vi "filter channels by name.vi"(10 "allowed name patterns":string[](array[string]), 11 "channels in":refnum<class "TBM channel.lvclass">[](array[class])) -> (3 "channels out":refnum<class "TBM channel.lvclass">[](array[class]))   [LabVIEW 2013, in "TBM channel.lvclass"]
doc: "Filters channels in based on their names and the list of allowed patterns. This function performs a simple pattern match for all <b>allowed name patterns</b> on each name from <b>channels in</b>"
uses:
  TBM channel.lvclass
  <vilib>/NI/Tag Bus/tag/tag descriptor.lvclass/tag descriptor.ctl
  <vilib>/NI/Tag Bus/tag/tag descriptor.lvclass
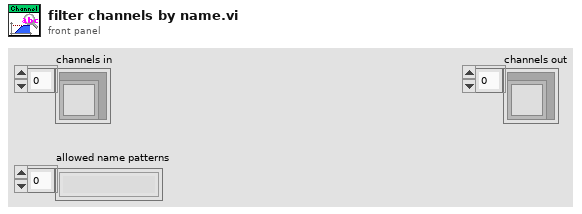
[diagram p1: front panel]
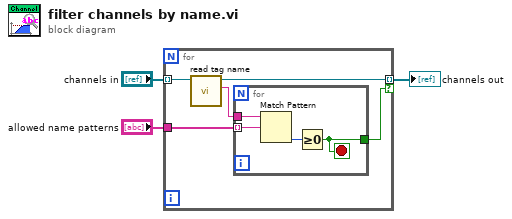
[diagram p0: block diagram]
diagram:
  n1 = for {
    tunnel: "channels in" -> [w8] mode=indexing
    tunnel: "allowed name patterns" -> [w5]
    tunnel: [w7] -> w1 mode=indexing if=w4
    n2 = call <vilib>:"read tag name.vi"("system tag in"=w8) -> ("name"=w6:string, "system tag out"=w7:refnum<class "TBM channel.lvclass">)  [unwired: 8 in, 1 out]
    n3 = for {
      tunnel: w6 -> [w12]
      tunnel: w5 -> [w11] mode=indexing
      tunnel: [w9] -> w4
      stop <- w9 stop-if-true
      n4 = Match Pattern(string=w12, regular expression=w11) -> (offset past match=w10:i32)  [unwired: 1 in, 3 out]
      n5 = Greater Or Equal To 0?(x=w10) -> (x >= 0?=w9:bool)
    }
  }
  "channels out" <- w1
